vi "LCDIO Get In Chan Handle.vi"(8 "error in (no error)":errorcluster caption="Fehler (Eingang, kein Fehler)", 11 "Index":u8) -> (0 "error out":errorcluster caption="Fehler (Ausgang)", 3 "Digital Input Channel":i64)   [LabVIEW 2021, in "labbCAN_DigIO_API.lvlib"]
doc: "LCDIO_Func long LCDIO_CALL LCDIO_GetInChanHandle(unsigned char Index,\n dev_hdl* pInChanHdl);"
uses:
  labbCAN_DigIO_API.lvlib
  labbCAN_DigIO_API.dll
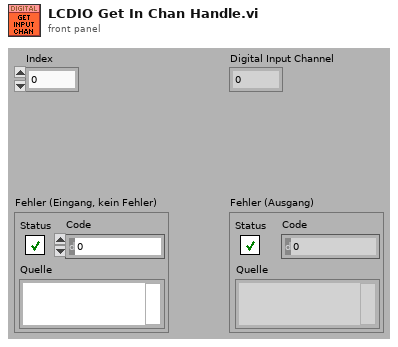
[diagram p1: front panel]
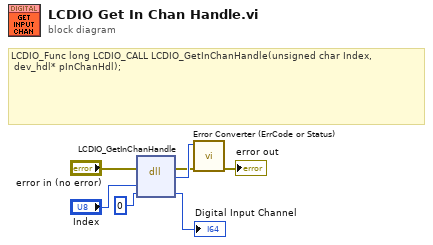
[diagram p0: block diagram]
diagram:
  # "LCDIO_Func long LCDIO_CALL LCDIO_GetInChanHandle(unsigned char Index,\n\tdev_hdl* pInChanHdl);"
  n1 = dll-call lib="C:/Users/olaja/AppData/Local/CETONI_SDK/labbCAN_DigIO_API.*" fn="LCDIO_GetInChanHandle"(error in="error in (no error)", "Index"="Index", "pInChanHdl"=i64 0) -> (error out=w3:errorcluster, "Rückgabetyp"=w7:i32, "pInChanHdl"=→"Digital Input Channel":i64)  [unwired: 3 in, 1 out]
  n2 = call "Error Converter (ErrCode or Status).vi"("error in (no error)"=w3, "error code"=w7) -> ("error out"=→"error out":errorcluster)  [unwired: 9 in]
